vi "ntr.flow-panel.update.vi"(9 "log cluster":T5 {"clk" format="%#.3f"}, 11 "Controls[]":refnum<vi>[](array[refnum])) -> ()   [LabVIEW 2024]
uses:
  controls/typeEngineLogCluster.ctl
  controls/type.StepFunction.ctl
  controls/UiCompactReport.ctl
  controls/Ui.nrt.flow-panel.ctl
  controls/UiNutritionFlowElement.ctl
  controls/type.nrt.elment-state.ctl
  controls/enum-ntr-io-format.ctl
  controls/UiScheduleTimestamp.ctl
  controls/UiNutritionPanel.ctl
panel:
  out "Missing Element?":bool
  out "State(Element)":string
  out "Elements Names":string[](array[string])
  in  "Unit Settings":T1={"WASH_IN"={"boolean"=FALSE, "Message"="25/150"}, "EC"={"boolean"=TRUE, "Message"="L Alarm"}, "PH"={"boolean"=TRUE, "Message"="Low"}, "ORP"={"boolean"=TRUE, "Message"="Range"}, "W_TEMP"={"boolean"=TRUE, "Message"="25"}, "W_LEVEL"={"boolean"=TRUE, "Message"="FULL"}, "ALFA1"={"boolean"=TRUE, "Message"="60/60"}, "BETA1"={"boolean"=TRUE, "Message"="25/60"}, "ALFA2"={"boolean"=FALSE, "Message"="0/0"}, "BETA2"={"boolean"=FALSE, "Message"="0/0"}, "ACID"={"boolean"=FALSE, "Message"="0/60"}, "BASE"={"boolean"=FALSE, "Message"="0/50"}, "WATER"={"boolean"=FALSE, "Message"="0/150"}, "WASH_OUT"={"boolean"=FALSE, "Message"="ss"}, "UNIT"={"boolean"=FALSE, "Message"="25/150"}, "ORPMIX"={"boolean"=FALSE, "Message"="0/150"}}
  in  "TEST VECTOR":T3[](array[typedef])=[{"ErrorFlag"=FALSE, "idx"=0, "Step Name"="", "Step Function"=enum."UNIT_CHECK", "Report"="UNIT1:Prepare for Sampling", "clk"=808.9115753173828, "Proc"=""}, {"ErrorFlag"=FALSE, "idx"=1, "Step Name"="_START_UNIT", "Step Function"=enum."_IO_WRITE", "Report"="UNVLV_1;1:143,", "clk"=809.013774394989, "Proc"=""}, {"ErrorFlag"=FALSE, "idx"=2, "Step Name"="_AUX", "Step Function"=enum."_IO_WRITE", "Report"="UNPMP_1;1:143,", "clk"=809.1302719116211, "Proc"=""}, {"ErrorFlag"=FALSE, "idx"=3, "Step Name"="_WASH_IN", "Step Function"=enum."_DELAY_LOAD", "Report"="3807441809", "clk"=809.2404737472534, "Proc"=""}, {"ErrorFlag"=FALSE, "idx"=4, "Step Name"="", "Step Function"=enum."_DELAY_COMPARE", "Report"="2.0/2.0", "clk"=811.2761874198914, "Proc"=""}, {"ErrorFlag"=FALSE, "idx"=5, "Step Name"="", "Step Function"=enum."UNIT_SAMPLE", "Report"="UNIT=1;EC=2.7 LOW;PH=-38.0 ALARM;ORP=-38.0 ALARM;UNWL_1=0.0 LOW", "clk"=841.9652895927429, "Proc"=""}, {"ErrorFlag"=FALSE, "idx"=6, "Step Name"="", "Step Function"=enum."UNIT_DOSE", "Report"="pump=ALFA1;dose=2;counter=62;limit=200", "clk"=842.2391471862793, "Proc"=""}, {"ErrorFlag"=FALSE, "idx"=7, "Step Name"="_START_ALFA1", "Step Function"=enum."_IO_WRITE", "Report"="ALFA1;1:2,", "clk"=842.3526463508606, "Proc"=""}, {"ErrorFlag"=FALSE, "idx"=8, "Step Name"="_WAIT_ALFA1", "Step Function"=enum."_DELAY_LOAD", "Report"="3807441842", "clk"=842.4676065444946, "Proc"=""}, {"ErrorFlag"=FALSE, "idx"=9, "Step Name"="", "Step Function"=enum."_DELAY_COMPARE", "Report"="2.1/2.0", "clk"=844.5177793502808, "Proc"=""}, {"ErrorFlag"=FALSE, "idx"=10, "Step Name"="", "Step Function"=enum."UNIT_DOSE", "Report"="pump=BETA1;dose=2;counter=42;limit=100", "clk"=844.6215801239014, "Proc"=""}, {"ErrorFlag"=FALSE, "idx"=11, "Step Name"="_START_BETA1", "Step Function"=enum."_IO_WRITE", "Report"="BETA1;1:2,", "clk"=844.7354688644409, "Proc"=""}, {"ErrorFlag"=FALSE, "idx"=12, "Step Name"="_WAIT_BETA1", "Step Function"=enum."_DELAY_LOAD", "Report"="3807441845", "clk"=844.8503303527832, "Proc"=""}, {"ErrorFlag"=FALSE, "idx"=13, "Step Name"="", "Step Function"=enum."_DELAY_COMPARE", "Report"="2.1/2.0", "clk"=846.9136576652527, "Proc"=""}, {"ErrorFlag"=FALSE, "idx"=14, "Step Name"="", "Step Function"=enum."UNIT_DOSE", "Report"="pump=ALFA2;dose=3;counter=0;limit=20", "clk"=847.0166110992432, "Proc"=""}, {"ErrorFlag"=FALSE, "idx"=15, "Step Name"="_START_ALFA2", "Step Function"=enum."_IO_WRITE", "Report"="ALFA2;1:3,", "clk"=847.1284127235413, "Proc"=""}, {"ErrorFlag"=FALSE, "idx"=16, "Step Name"="_WAIT_ALFA2", "Step Function"=enum."_DELAY_LOAD", "Report"="3807441847", "clk"=847.2391495704651, "Proc"=""}, {"ErrorFlag"=FALSE, "idx"=17, "Step Name"="", "Step Function"=enum."_DELAY_COMPARE", "Report"="3.0/3.0", "clk"=850.2459425926208, "Proc"=""}, {"ErrorFlag"=FALSE, "idx"=18, "Step Name"="", "Step Function"=enum."UNIT_DOSE", "Report"="pump=BETA2;dose=3;counter=0;limit=20", "clk"=850.34832239151, "Proc"=""}, {"ErrorFlag"=FALSE, "idx"=19, "Step Name"="_START_BETA2", "Step Function"=enum."_IO_WRITE", "Report"="BETA2;1:3,", "clk"=850.4585151672363, "Proc"=""}, {"ErrorFlag"=FALSE, "idx"=20, "Step Name"="_WAIT_BETA2", "Step Function"=enum."_DELAY_LOAD", "Report"="3807441851", "clk"=850.5737953186035, "Proc"=""}, {"ErrorFlag"=FALSE, "idx"=21, "Step Name"="", "Step Function"=enum."_DELAY_COMPARE", "Report"="3.0/3.0", "clk"=853.5802583694458, "Proc"=""}, {"ErrorFlag"=FALSE, "idx"=22, "Step Name"="_WATER_AUX_OFF", "Step Function"=enum."_IO_WRITE", "Report"="UNPMP_1;0:0,", "clk"=853.6832575798035, "Proc"=""}, {"ErrorFlag"=FALSE, "idx"=23, "Step Name"="", "Step Function"=enum."UNIT_DOSE", "Report"="pump=WATER;dose=2;counter=20;limit=100", "clk"=853.7997298240662, "Proc"=""}, {"ErrorFlag"=FALSE, "idx"=24, "Step Name"="_START_WATER", "Step Function"=enum."_IO_WRITE", "Report"="WATER;1:2,", "clk"=853.9108262062073, "Proc"=""}, {"ErrorFlag"=FALSE, "idx"=25, "Step Name"="_WAIT_WATER", "Step Function"=enum."_DELAY_LOAD", "Report"="3807441854", "clk"=854.0239872932434, "Proc"=""}, {"ErrorFlag"=FALSE, "idx"=26, "Step Name"="", "Step Function"=enum."_DELAY_COMPARE", "Report"="2.1/2.0", "clk"=856.0921583175659, "Proc"=""}, {"ErrorFlag"=FALSE, "idx"=27, "Step Name"="_STOP_UNIT", "Step Function"=enum."_IO_WRITE", "Report"="UNVLV_1;0:0,", "clk"=856.1950078010559, "Proc"=""}, {"ErrorFlag"=FALSE, "idx"=28, "Step Name"="_AUX", "Step Function"=enum."_IO_WRITE", "Report"="UNPMP_1;0:0,", "clk"=856.3099999427795, "Proc"=""}, {"ErrorFlag"=FALSE, "idx"=29, "Step Name"="", "Step Function"=enum."UNIT_CHECK", "Report"="UNIT2:Unit Disabled", "clk"=856.4237542152405, "Proc"=""}, {"ErrorFlag"=FALSE, "idx"=30, "Step Name"="CYCLE_INTERVAL", "Step Function"=enum."_DELAY_LOAD", "Report"="3807441857", "clk"=856.5289416313171, "Proc"=""}, {"ErrorFlag"=FALSE, "idx"=31, "Step Name"="", "Step Function"=enum."_DELAY_COMPARE", "Report"="2.9/3.0", "clk"=859.4704394340515, "Proc"=""}] {"clk" format="%#.1f"}
  out "result string":string
  out "Step Name":string
  out "State":string
  in  "appended array":T5[](array[typedef])=[{"Proc Name"="NUTRITION", "ProcPath"="", "Step Name"="", "Step Function"=enum."_DELAY_COMPARE", "Step Index"=9, "Report"="1.5/3.0", "clk"=3806463695.106538, "error in"={"status"=FALSE, "code"=0, "source"=""}, "Log Message"="", "Proc Module"=""}, {"Proc Name"="NUTRITION", "ProcPath"="", "Step Name"="", "Step Function"=enum."_DELAY_COMPARE", "Step Index"=9, "Report"="0.8/3.0", "clk"=3806463694.341048, "error in"={"status"=FALSE, "code"=0, "source"=""}, "Log Message"="", "Proc Module"=""}, {"Proc Name"="NUTRITION", "ProcPath"="", "Step Name"="_WAIT_ALFA1", "Step Function"=enum."_DELAY_LOAD", "Step Index"=8, "Report"="", "clk"=3806463693.5845046, "error in"={"status"=FALSE, "code"=0, "source"=""}, "Log Message"="", "Proc Module"=""}, {"Proc Name"="NUTRITION", "ProcPath"="", "Step Name"="_AUX", "Step Function"=enum."_IO_WRITE", "Step Index"=7, "Report"="UNIT1,1:3,", "clk"=3806463692.8226175, "error in"={"status"=FALSE, "code"=0, "source"=""}, "Log Message"="", "Proc Module"=""}, {"Proc Name"="NUTRITION", "ProcPath"="", "Step Name"="_START_ALFA1", "Step Function"=enum."_IO_WRITE", "Step Index"=6, "Report"="ALFA1,1:3,", "clk"=3806463692.024861, "error in"={"status"=FALSE, "code"=0, "source"=""}, "Log Message"="", "Proc Module"=""}, {"Proc Name"="NUTRITION", "ProcPath"="", "Step Name"="", "Step Function"=enum."UNIT_DOSE", "Step Index"=5, "Report"="pump=ALFA1;dose=3;counter=3;limit=15", "clk"=3806463691.2188854, "error in"={"status"=FALSE, "code"=0, "source"=""}, "Log Message"="", "Proc Module"=""}, {"Proc Name"="NUTRITION", "ProcPath"="", "Step Name"="", "Step Function"=enum."UNIT_SAMPLE", "Step Index"=4, "Report"="UNIT=1;EC=5.0_LOW;PH=0.0_ALARM;ORP=-99;W_LEVEL=FULL;W_TEMP=25", "clk"=3806463690.4068866, "error in"={"status"=FALSE, "code"=0, "source"=""}, "Log Message"="", "Proc Module"=""}, {"Proc Name"="NUTRITION", "ProcPath"="", "Step Name"="", "Step Function"=enum."_DELAY_COMPARE", "Step Index"=3, "Report"="0.3/0.0", "clk"=3806463682.7784977, "error in"={"status"=FALSE, "code"=0, "source"=""}, "Log Message"="", "Proc Module"=""}, {"Proc Name"="NUTRITION", "ProcPath"="", "Step Name"="_WASH_IN", "Step Function"=enum."_DELAY_LOAD", "Step Index"=2, "Report"="", "clk"=3806463682.5215073, "error in"={"status"=FALSE, "code"=0, "source"=""}, "Log Message"="", "Proc Module"=""}, {"Proc Name"="NUTRITION", "ProcPath"="", "Step Name"="_START_FLOW", "Step Function"=enum."_IO_WRITE", "Step Index"=1, "Report"="UNIT1,1:5,", "clk"=3806463682.2498655, "error in"={"status"=FALSE, "code"=0, "source"=""}, "Log Message"="", "Proc Module"=""}, {"Proc Name"="NUTRITION", "ProcPath"="", "Step Name"="", "Step Function"=enum."UNIT_CHECK", "Step Index"=0, "Report"="UNIT1", "clk"=3806463681.9819593, "error in"={"status"=FALSE, "code"=0, "source"=""}, "Log Message"="", "Proc Module"=""}, {"Proc Name"="NUTRITION", "ProcPath"="", "Step Name"="", "Step Function"=enum."UNIT_CHECK", "Step Index"=0, "Report"="UNIT1", "clk"=3806457099.490219, "error in"={"status"=FALSE, "code"=0, "source"=""}, "Log Message"="", "Proc Module"=""}, {"Proc Name"="NUTRITION", "ProcPath"="", "Step Name"="_START_FLOW", "Step Function"=enum."_IO_WRITE", "Step Index"=1, "Report"="UNIT1,1:5,", "clk"=3806457099.753702, "error in"={"status"=FALSE, "code"=0, "source"=""}, "Log Message"="", "Proc Module"=""}, {"Proc Name"="NUTRITION", "ProcPath"="", "Step Name"="_WASH_IN", "Step Function"=enum."_DELAY_LOAD", "Step Index"=2, "Report"="", "clk"=3806457100.018482, "error in"={"status"=FALSE, "code"=0, "source"=""}, "Log Message"="", "Proc Module"=""}, {"Proc Name"="NUTRITION", "ProcPath"="", "Step Name"="", "Step Function"=enum."_DELAY_COMPARE", "Step Index"=3, "Report"="0.3/0.0", "clk"=3806457100.2720094, "error in"={"status"=FALSE, "code"=0, "source"=""}, "Log Message"="", "Proc Module"=""}, {"Proc Name"="NUTRITION", "ProcPath"="", "Step Name"="", "Step Function"=enum."UNIT_SAMPLE", "Step Index"=4, "Report"="UNIT=1;EC=5.0_LOW;PH=0.0_ALARM;ORP=-99;W_LEVEL=FULL;W_TEMP=25", "clk"=3806457100.531534, "error in"={"status"=FALSE, "code"=0, "source"=""}, "Log Message"="", "Proc Module"=""}, {"Proc Name"="NUTRITION", "ProcPath"="", "Step Name"="", "Step Function"=enum."UNIT_DOSE", "Step Index"=5, "Report"="ALFA1:3_0/15", "clk"=3806457100.830936, "error in"={"status"=FALSE, "code"=0, "source"=""}, "Log Message"="", "Proc Module"=""}, {"Proc Name"="NUTRITION", "ProcPath"="", "Step Name"="_START_ALFA1", "Step Function"=enum."_IO_WRITE", "Step Index"=6, "Report"="ALFA1,1:3,", "clk"=3806457101.096012, "error in"={"status"=FALSE, "code"=0, "source"=""}, "Log Message"="", "Proc Module"=""}, {"Proc Name"="NUTRITION", "ProcPath"="", "Step Name"="_AUX", "Step Function"=enum."_IO_WRITE", "Step Index"=7, "Report"="UNIT1,1:3,", "clk"=3806457101.359422, "error in"={"status"=FALSE, "code"=0, "source"=""}, "Log Message"="", "Proc Module"=""}, {"Proc Name"="NUTRITION", "ProcPath"="", "Step Name"="_WAIT_ALFA1", "Step Function"=enum."_DELAY_LOAD", "Step Index"=8, "Report"="", "clk"=3806457101.636155, "error in"={"status"=FALSE, "code"=0, "source"=""}, "Log Message"="", "Proc Module"=""}, {"Proc Name"="NUTRITION", "ProcPath"="", "Step Name"="", "Step Function"=enum."_DELAY_COMPARE", "Step Index"=9, "Report"="0.3/3.0", "clk"=3806457101.890099, "error in"={"status"=FALSE, "code"=0, "source"=""}, "Log Message"="", "Proc Module"=""}, {"Proc Name"="NUTRITION", "ProcPath"="", "Step Name"="", "Step Function"=enum."_DELAY_COMPARE", "Step Index"=9, "Report"="0.5/3.0", "clk"=3806457102.145725, "error in"={"status"=FALSE, "code"=0, "source"=""}, "Log Message"="", "Proc Module"=""}, {"Proc Name"="NUTRITION", "ProcPath"="", "Step Name"="", "Step Function"=enum."_DELAY_COMPARE", "Step Index"=9, "Report"="0.8/3.0", "clk"=3806457102.4017487, "error in"={"status"=FALSE, "code"=0, "source"=""}, "Log Message"="", "Proc Module"=""}, {"Proc Name"="NUTRITION", "ProcPath"="", "Step Name"="", "Step Function"=enum."_DELAY_COMPARE", "Step Index"=9, "Report"="1.0/3.0", "clk"=3806457102.662003, "error in"={"status"=FALSE, "code"=0, "source"=""}, "Log Message"="", "Proc Module"=""}, {"Proc Name"="NUTRITION", "ProcPath"="", "Step Name"="", "Step Function"=enum."_DELAY_COMPARE", "Step Index"=9, "Report"="1.3/3.0", "clk"=3806457102.9161887, "error in"={"status"=FALSE, "code"=0, "source"=""}, "Log Message"="", "Proc Module"=""}, {"Proc Name"="NUTRITION", "ProcPath"="", "Step Name"="", "Step Function"=enum."_DELAY_COMPARE", "Step Index"=9, "Report"="1.5/3.0", "clk"=3806457103.1737394, "error in"={"status"=FALSE, "code"=0, "source"=""}, "Log Message"="", "Proc Module"=""}, {"Proc Name"="NUTRITION", "ProcPath"="", "Step Name"="", "Step Function"=enum."_DELAY_COMPARE", "Step Index"=9, "Report"="1.8/3.0", "clk"=3806457103.4284744, "error in"={"status"=FALSE, "code"=0, "source"=""}, "Log Message"="", "Proc Module"=""}, {"Proc Name"="NUTRITION", "ProcPath"="", "Step Name"="", "Step Function"=enum."_DELAY_COMPARE", "Step Index"=9, "Report"="2.0/3.0", "clk"=3806457103.683892, "error in"={"status"=FALSE, "code"=0, "source"=""}, "Log Message"="", "Proc Module"=""}, {"Proc Name"="NUTRITION", "ProcPath"="", "Step Name"="", "Step Function"=enum."_DELAY_COMPARE", "Step Index"=9, "Report"="2.3/3.0", "clk"=3806457103.9400506, "error in"={"status"=FALSE, "code"=0, "source"=""}, "Log Message"="", "Proc Module"=""}, {"Proc Name"="NUTRITION", "ProcPath"="", "Step Name"="", "Step Function"=enum."_DELAY_COMPARE", "Step Index"=9, "Report"="2.6/3.0", "clk"=3806457104.203483, "error in"={"status"=FALSE, "code"=0, "source"=""}, "Log Message"="", "Proc Module"=""}, {"Proc Name"="NUTRITION", "ProcPath"="", "Step Name"="", "Step Function"=enum."_DELAY_COMPARE", "Step Index"=9, "Report"="2.8/3.0", "clk"=3806457104.4665594, "error in"={"status"=FALSE, "code"=0, "source"=""}, "Log Message"="", "Proc Module"=""}, {"Proc Name"="NUTRITION", "ProcPath"="", "Step Name"="", "Step Function"=enum."_DELAY_COMPARE", "Step Index"=9, "Report"="3.1/3.0", "clk"=3806457104.722045, "error in"={"status"=FALSE, "code"=0, "source"=""}, "Log Message"="", "Proc Module"=""}, {"Proc Name"="NUTRITION", "ProcPath"="", "Step Name"="", "Step Function"=enum."UNIT_DOSE", "Step Index"=10, "Report"="BETA1:3_0/15", "clk"=3806457104.9829454, "error in"={"status"=FALSE, "code"=0, "source"=""}, "Log Message"="", "Proc Module"=""}, {"Proc Name"="NUTRITION", "ProcPath"="", "Step Name"="_START_BETA1", "Step Function"=enum."_IO_WRITE", "Step Index"=11, "Report"="BETA1,1:3,", "clk"=3806457105.259259, "error in"={"status"=FALSE, "code"=0, "source"=""}, "Log Message"="", "Proc Module"=""}, {"Proc Name"="NUTRITION", "ProcPath"="", "Step Name"="_AUX", "Step Function"=enum."_IO_WRITE", "Step Index"=12, "Report"="UNIT1,1:3,", "clk"=3806457105.5364633, "error in"={"status"=FALSE, "code"=0, "source"=""}, "Log Message"="", "Proc Module"=""}, {"Proc Name"="NUTRITION", "ProcPath"="", "Step Name"="_WAIT_BETA1", "Step Function"=enum."_DELAY_LOAD", "Step Index"=13, "Report"="", "clk"=3806457105.8045793, "error in"={"status"=FALSE, "code"=0, "source"=""}, "Log Message"="", "Proc Module"=""}, {"Proc Name"="NUTRITION", "ProcPath"="", "Step Name"="", "Step Function"=enum."_DELAY_COMPARE", "Step Index"=14, "Report"="0.3/3.0", "clk"=3806457106.0651937, "error in"={"status"=FALSE, "code"=0, "source"=""}, "Log Message"="", "Proc Module"=""}, {"Proc Name"="NUTRITION", "ProcPath"="", "Step Name"="", "Step Function"=enum."_DELAY_COMPARE", "Step Index"=14, "Report"="0.5/3.0", "clk"=3806457106.321509, "error in"={"status"=FALSE, "code"=0, "source"=""}, "Log Message"="", "Proc Module"=""}] {"clk" format="%#.3f"}
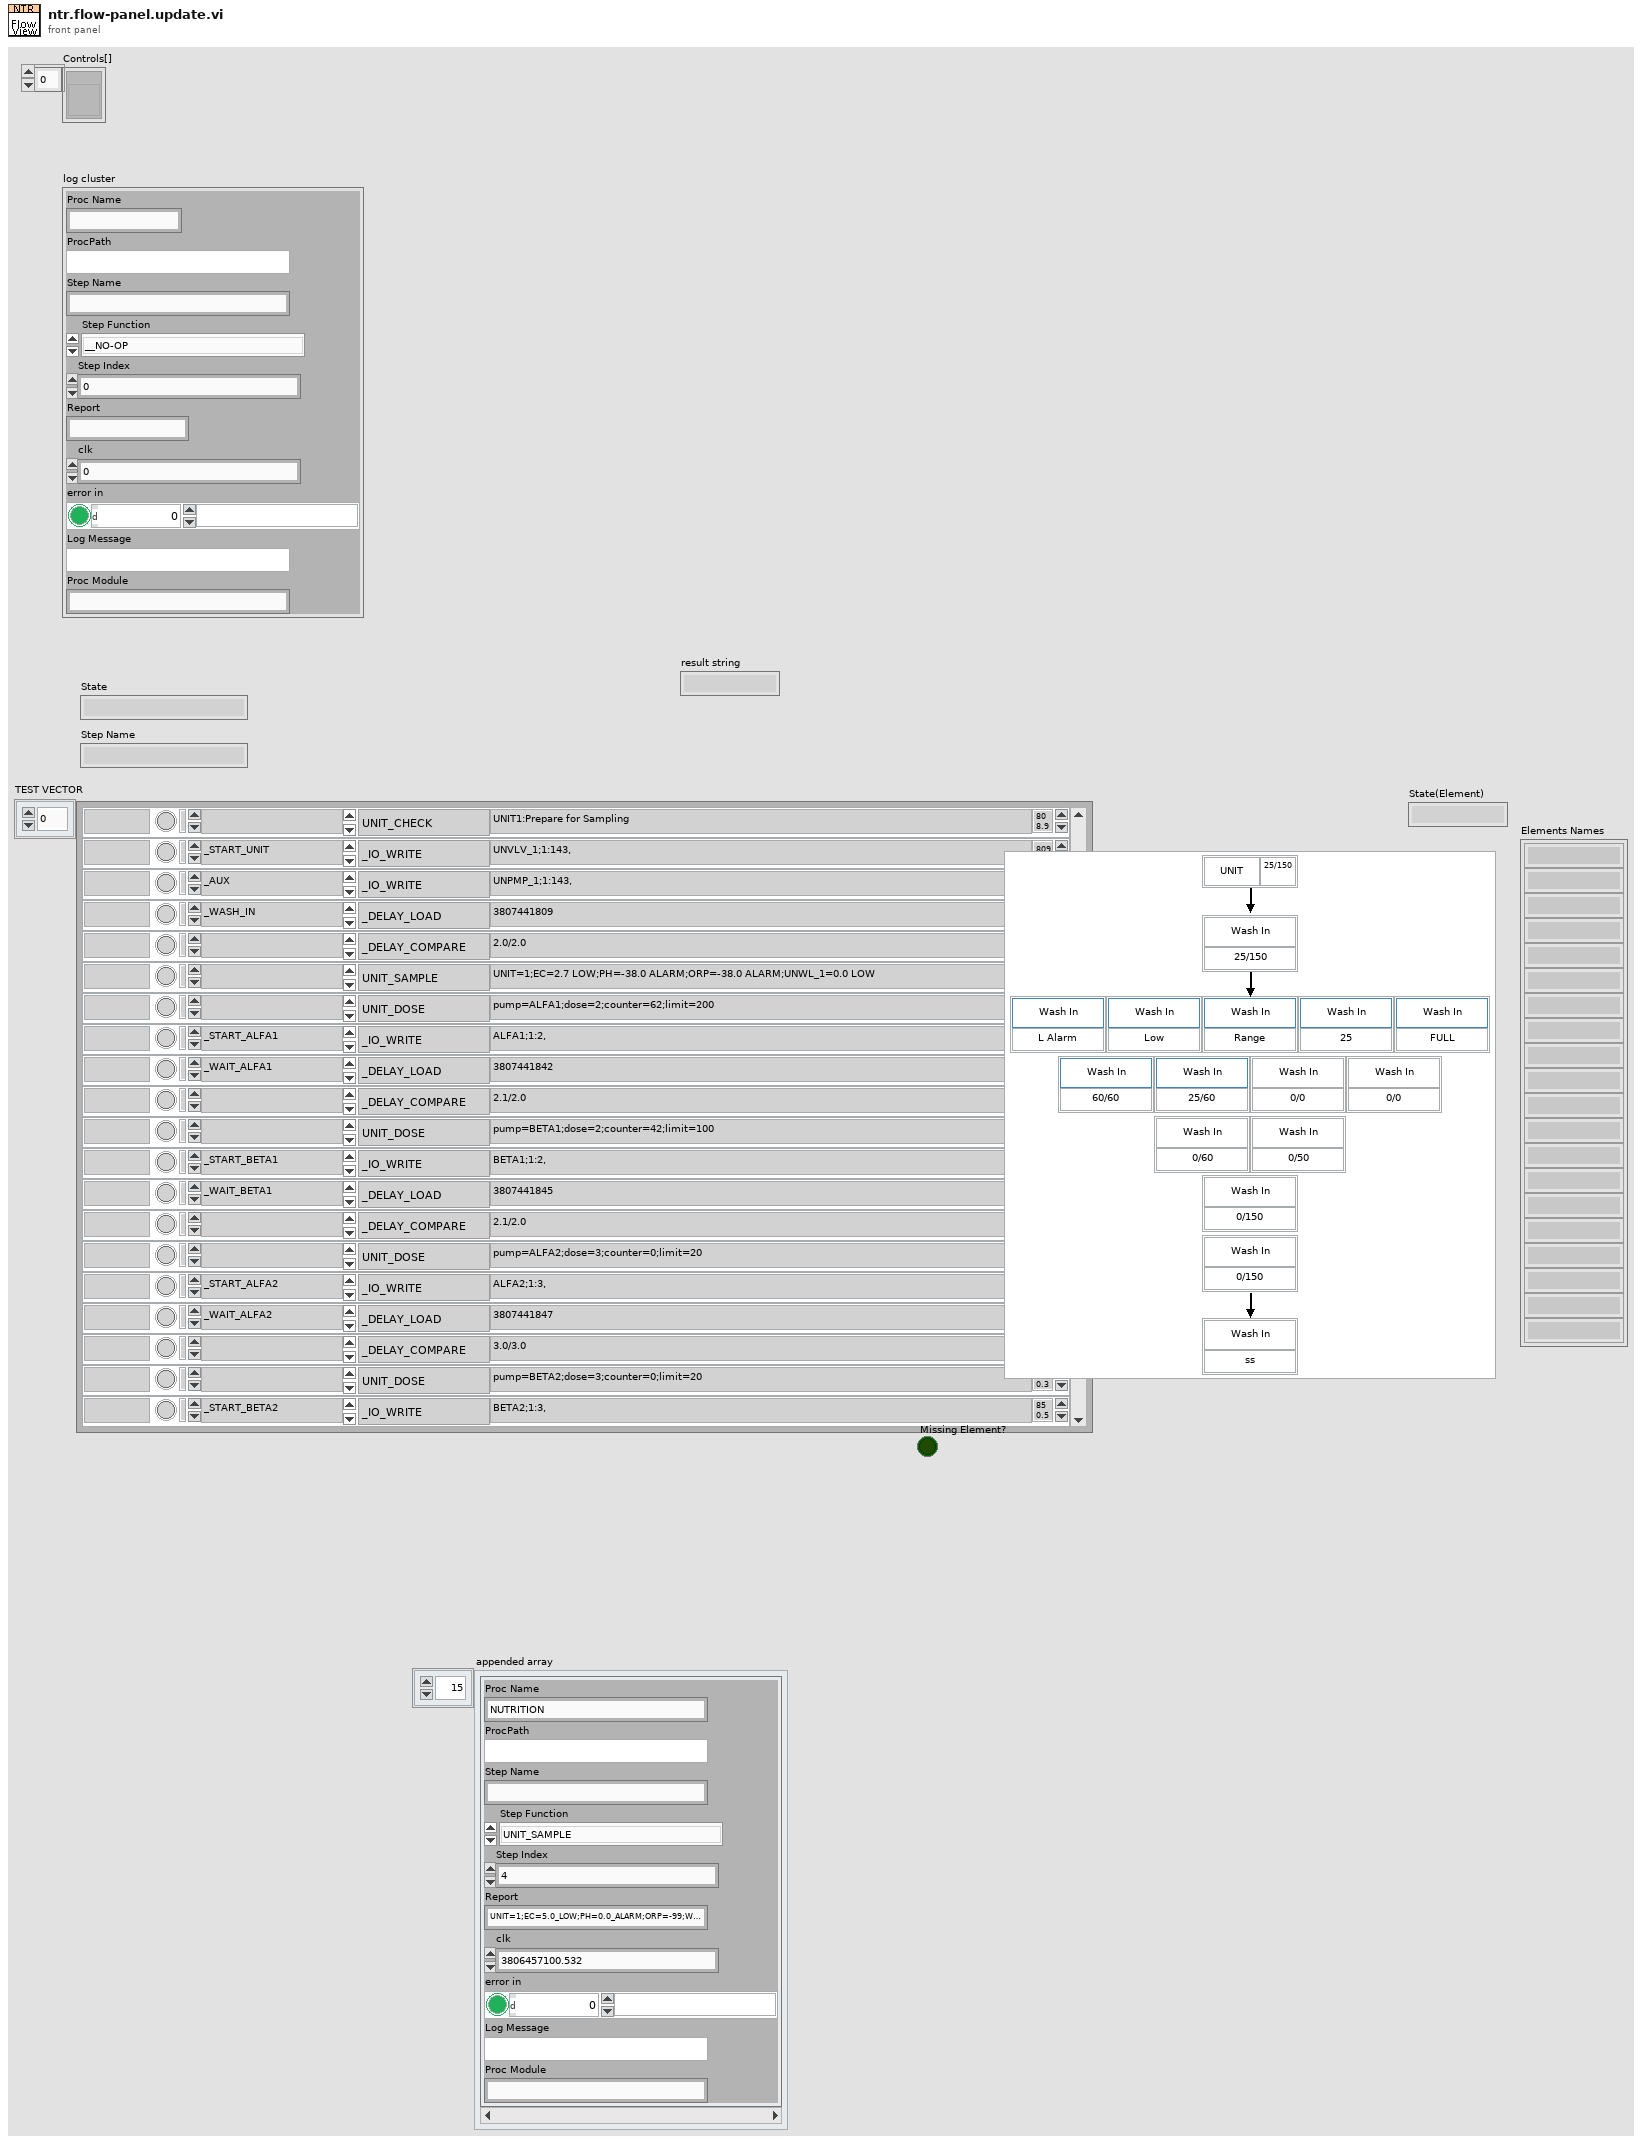
[diagram p1: front panel]
types:
  T1 = typedef "Ui.nrt.flow-panel.ctl" = cluster{"WASH_IN":T2, "EC":T2, "PH":T2, "ORP":T2, "W_TEMP":T2, "W_LEVEL":T2, "ALFA1":T2, "BETA1":T2, "ALFA2":T2, "BETA2":T2, "ACID":T2, "BASE":T2, "WATER":T2, "WASH_OUT":T2, "UNIT":cluster{"boolean":bool, "Message":string}, "ORPMIX":T2}
  T2 = typedef "UiNutritionFlowElement.ctl" = cluster{"boolean":bool, "Message":string}
  T3 = typedef "UiCompactReport.ctl" = cluster{"ErrorFlag":bool, "idx":i32, "Step Name":string, "Step Function":T4, "Report":string, "clk":dbl, "Proc":string}
  T4 = typedef "type.StepFunction.ctl" = enum16{"__NO-OP", "_DELAY_LOAD", "_DELAY_COMPARE", "_JUMP", "_COMPLETE", "_COMPARE", "_LOG_MESSAGE", "_LOG_LAST_REPORT", "_SCHEDULE", "_SCHED_DAILY", "CLK_COMPARE", "PROC_START", "PROC_STOP", "PROC_LOAD", "PROC_COMPLETION_CHECK", "PROC_COMPLETION_LOAD", "_IO_READ", "_IO_READ_MANY", "_IO_WRITE", "_IO_WRITE_BY_REG", "_IO_GET_OUTPUT", "_OCS_CHECK", "_OCS_RECORD", "_GET_RH", "_GET_ACC_UV", "_GET_WD", "_GET_WS", "_REC_DELETE", "_REC_MOVE", "_REC_COPY", "_IRR_CHECK", "UNIT_CHECK", "UNIT_SAMPLE", "UNIT_DOSE"}
  T5 = typedef "typeEngineLogCluster.ctl" = cluster{"Proc Name":string, "ProcPath":string, "Step Name":string, "Step Function":T4, "Step Index":i32, "Report":string, "clk":dbl, "error in":errorcluster, "Log Message":string, "Proc Module":string}
  T6 = typedef "type.nrt.elment-state.ctl" = enum16{"No Change", "OFF", "In Range", "Out of Range", "Alarm"}
  T7 = typedef "UiNutritionPanel.ctl" = cluster{"Main":cluster{"Enable":bool, "WashTimes":cluster{"In":dbl, "Out":dbl}, "DailyActivityHours":cluster{"Begin Time":T8, "End Time":T8}[]}, "Water Dosing":cluster{"Water Dose":dbl, "Water Limit":dbl}, "EC Ranges":cluster{"H Alarm":dbl, "L Alarm":dbl, "Low":dbl}, "EC Dosing":cluster{"ALFA1 Dose":dbl, "ALFA1 Limit":dbl, "BETA1 Dose":dbl, "BETA1 Limit":dbl, "ALFA2 Dose":dbl, "ALFA2 Limit":dbl, "BETA2 Dose":dbl, "BETA2 Limit":dbl}, "PH Ranges":cluster{"H Alarm":dbl, "L Alarm":dbl, "High":dbl, "Low":dbl}, "PH Dosing":cluster{"ACID Dose":dbl, "ACID Limit":dbl, "BASE Dose":dbl, "BASE Limit":dbl}, "ORP Ranges":cluster{"H Alarm":dbl, "L Alarm":dbl, "Low":dbl}, "ORP Dosing":cluster{"MIX Dose":dbl, "MIX Limit":dbl}}
  T8 = typedef "UiScheduleTimestamp.ctl" = timestamp
  T9 = typedef "enum-ntr-io-format.ctl" = enum16{"UN_VLV%d", "UN_PMP%d", "UN_WL%d", "UN_PH", "UN_EC", "UN_ORP", "UN_WT", "UN_PH2", "UN_ALFA1", "UN_BETA1", "UN_ALFA2", "UN_BETA2", "UN_ACID", "UN_BASE", "UN_WATER", "UN_ORPMIX"}
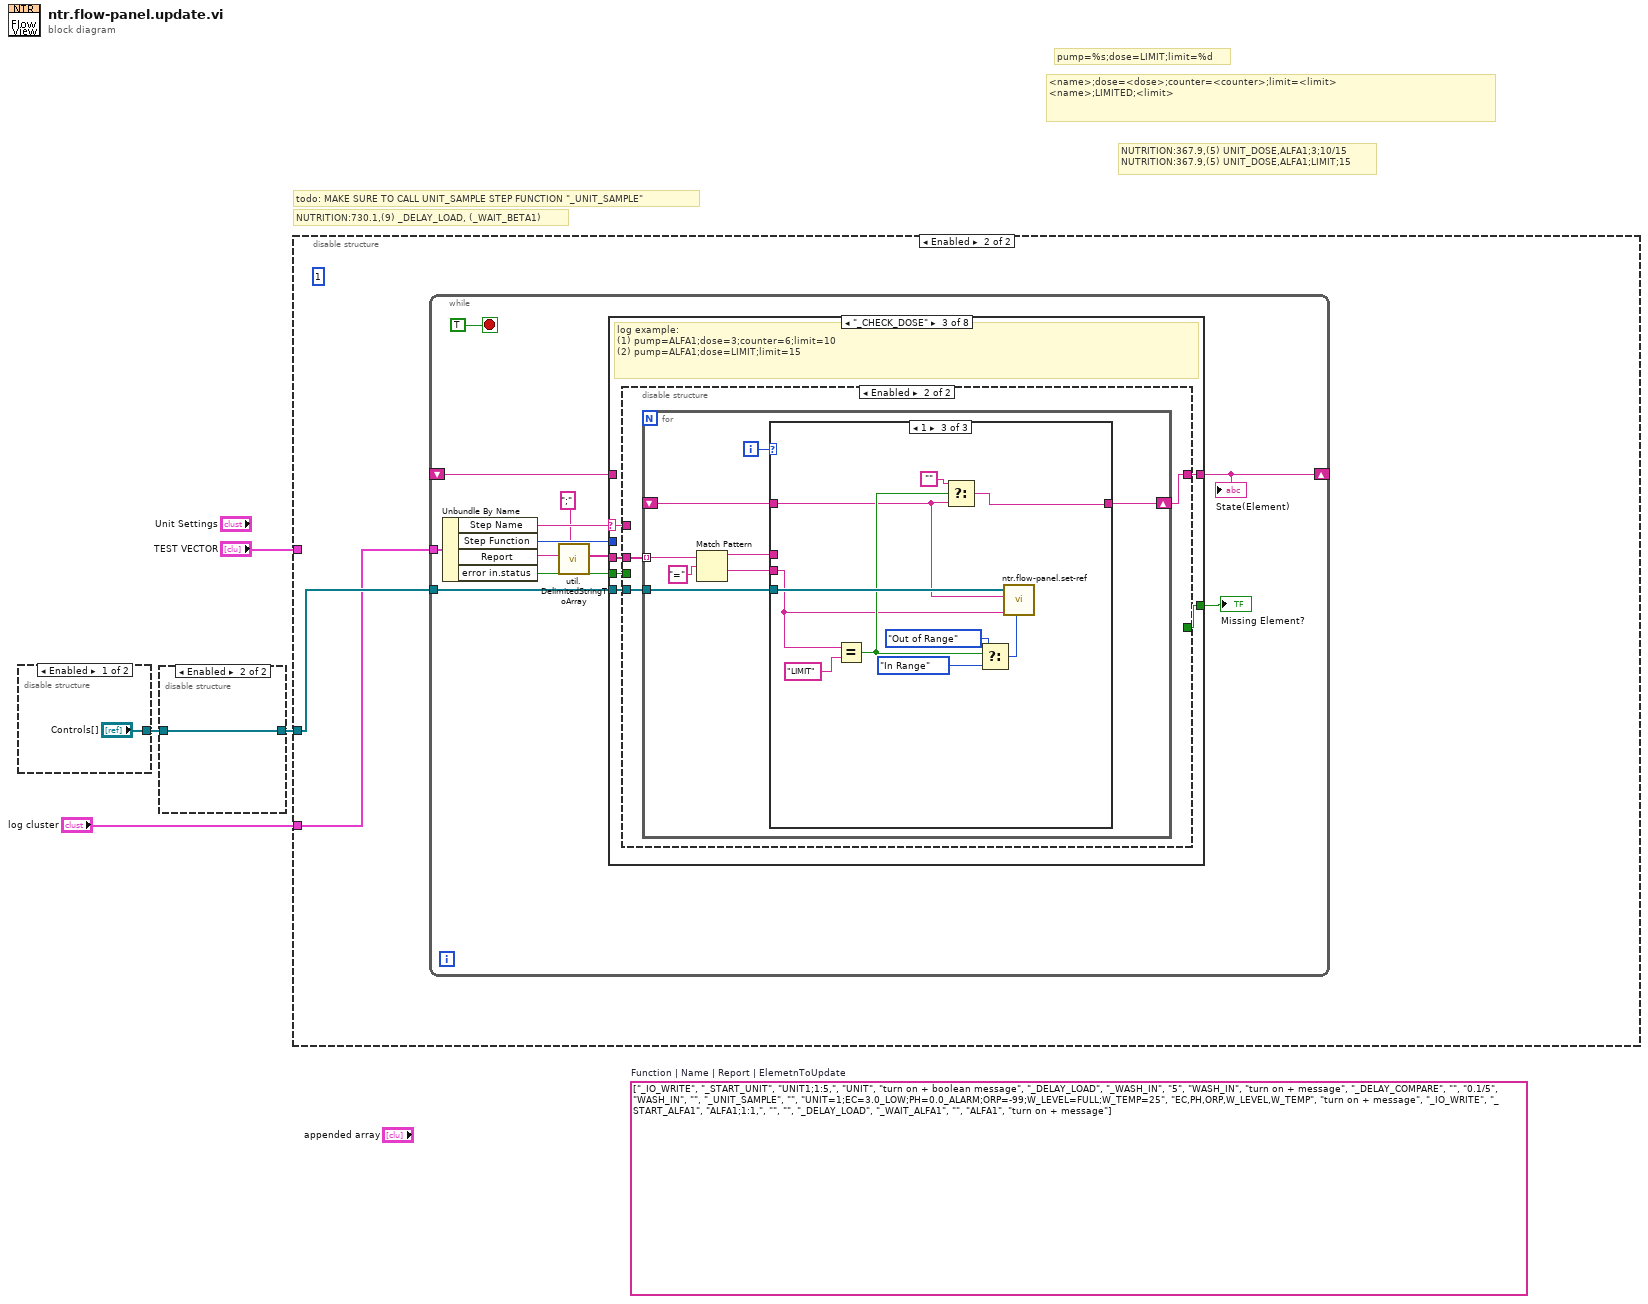
[diagram p0: block diagram]
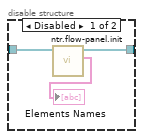
[diagram p2: hidden frame]
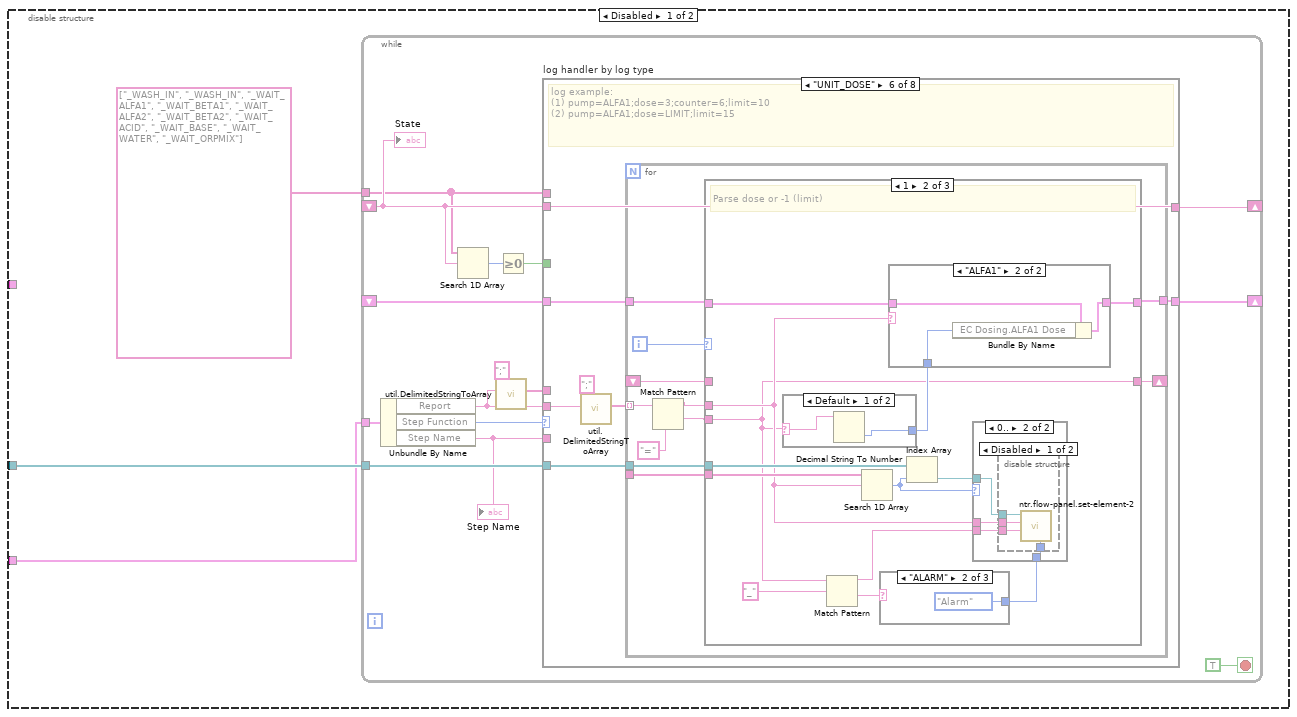
[diagram p3: hidden frame]
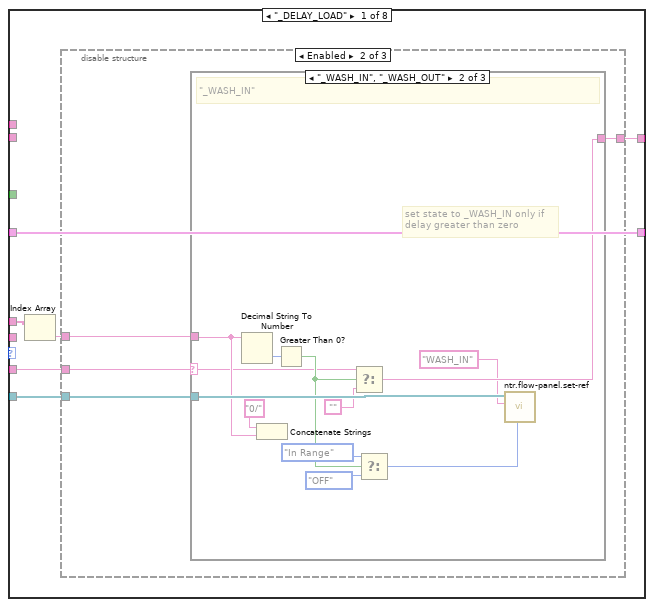
[diagram p4: hidden frame]
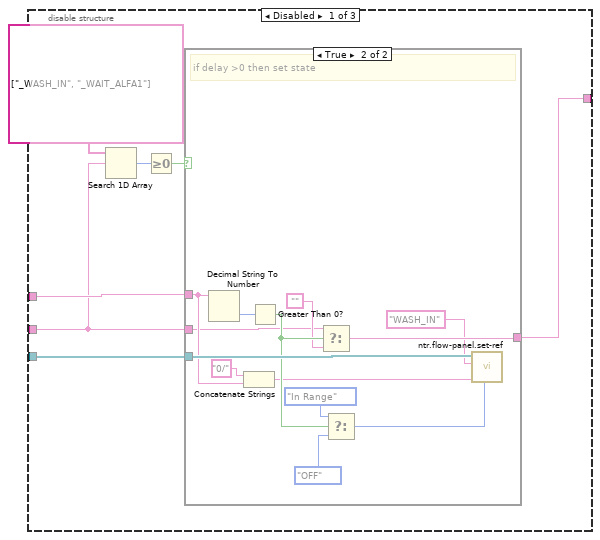
[diagram p5: hidden frame]
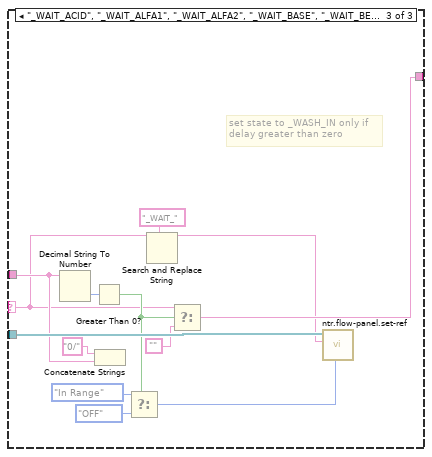
[diagram p8: hidden frame]
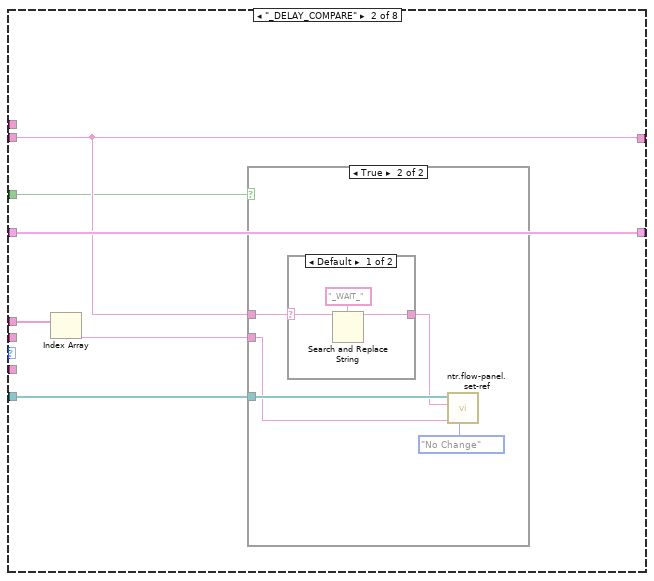
[diagram p10: hidden frame]
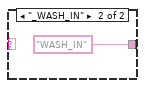
[diagram p12: hidden frame]
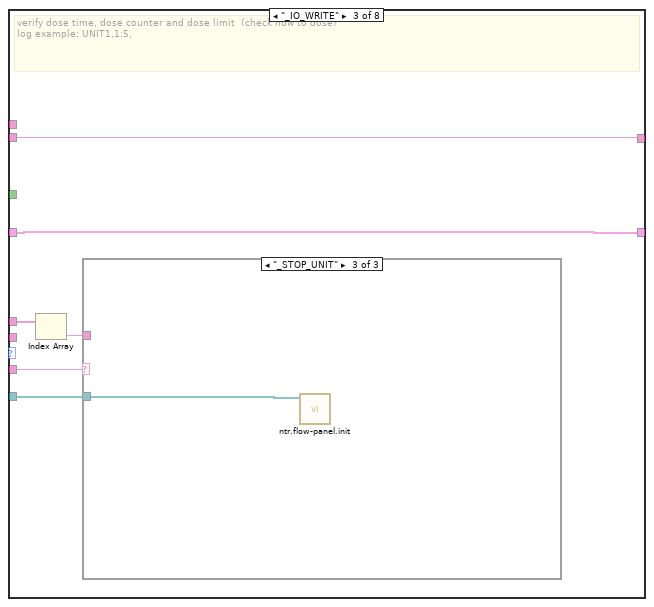
[diagram p13: hidden frame]
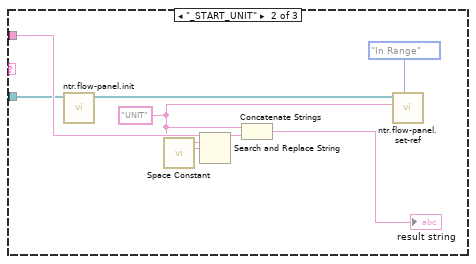
[diagram p15: hidden frame]
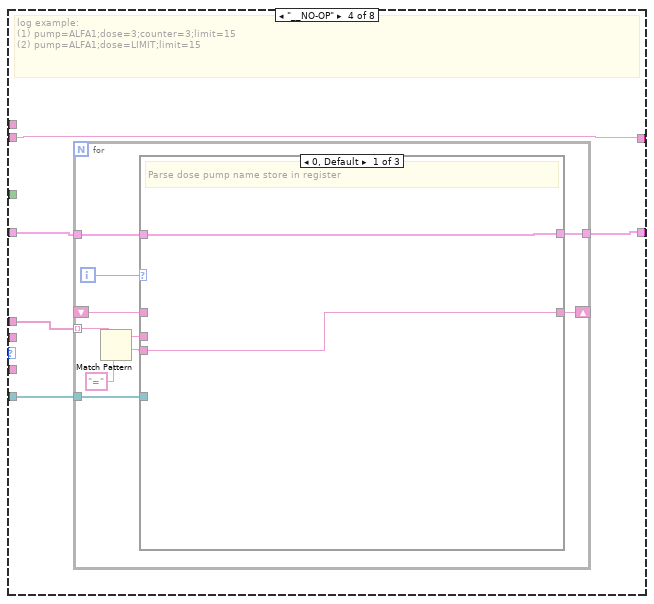
[diagram p16: hidden frame]
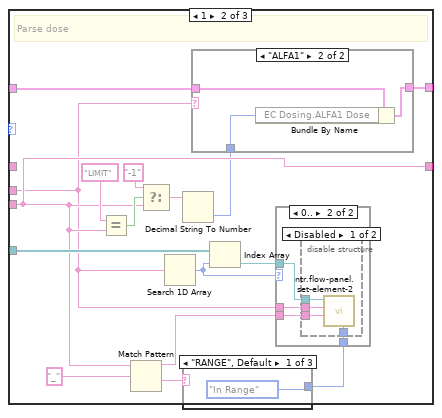
[diagram p17: hidden frame]
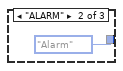
[diagram p19: hidden frame]
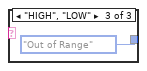
[diagram p20: hidden frame]
diagram:
  (unwired) string[][] [["_IO_WRITE", "_START_UNIT", "UNIT1;1:5,", "UNIT", "turn on + boolean message"], ["_DELAY_LOAD", "_WASH_IN", "5", "WASH_IN", "turn on + message"], ["_DELAY_COMPARE", "", "0.1/5", "WASH_IN", ""], ["_UNIT_SAMPLE", "", "UNIT=1;EC=3.0_LOW;PH=0.0_ALARM;ORP=-99;W_LEVEL=FULL;W_TEMP=25", "EC,PH,ORP,W_LEVEL,W_TEMP", "turn on + message"], ["_IO_WRITE", "_START_ALFA1", "ALFA1;1:1,", "", ""], ["_DELAY_LOAD", "_WAIT_ALFA1", "", "ALFA1", "turn on + message"]]  # Function | Name | Report | ElemetnToUpdate
  # "todo: MAKE SURE TO CALL UNIT_SAMPLE STEP FUNCTION \"_UNIT_SAMPLE\""
  # "pump=%s;dose=LIMIT;limit=%d"
  # "NUTRITION:367.9,(5) UNIT_DOSE,ALFA1;3;10/15\nNUTRITION:367.9,(5) UNIT_DOSE,ALFA1;LIMIT;15"
  # "<name>;dose=<dose>;counter=<counter>;limit=<limit>\n<name>;LIMITED;<limit>"
  # "NUTRITION:730.1,(9) _DELAY_LOAD, (_WAIT_BETA1)"
  n1 = disable-structure shown="Enabled" {
    disable-tunnel: ["Controls[]" w6] -> w4
    frame Enabled {
    }
    frame Disabled {
      n2 = property on="Unit Settings" class="Clust (strict)"() -> ("Controls[]"=w6:refnum<vi>[])  [unwired: 2 in, 2 out]
    }
  }
  n3 = disable-structure shown="Enabled" {
    disable-tunnel: w4 -> [w9 w10]
    disable-tunnel: [w8 w10] -> w3
    frame Disabled {
      n4 = call "ntr.flow-panel.init.vi"("Controls in"=w9) -> ("Elements Names"=→"Elements Names":string[], "Controls out"=w8:refnum<vi>[])  [unwired: 8 in, 1 out]
    }
    frame Enabled {
    }
  }
  n5 = disable-structure shown="Enabled" {
    disable-tunnel: w3 -> [w13 w281]
    disable-tunnel: "TEST VECTOR" -> [_ _]
    disable-tunnel: "log cluster" -> [w11 w280]
    frame Disabled {
      n6 = while {
        tunnel: w13 -> [w28]
        tunnel: w11 -> [w27]
        shift-right: [w23] -> _
        shift-left: _ -> [w22]
        shift-right: [w18] -> _
        shift-left: _ -> [w17]
        tunnel: string[] ["_WASH_IN", "_WASH_IN", "_WAIT_ALFA1", "_WAIT_BETA1", "_WAIT_ALFA2", "_WAIT_BETA2", "_WAIT_ACID", "_WAIT_BASE", "_WAIT_WATER", "_WAIT_ORPMIX"] ("Element Name") -> [w14]
        stop <- TRUE stop-if-true
        n7 = Unbundle By Name(w27) -> ("Report"=w20:string, "Step Function"=w26:T4, "Step Name"=w25:string)
        "Step Name" <- w25
        n8 = Search 1D Array(1D array=w14, element=w17) -> (index of element=w16:i32)  [unwired: 1 in]
        n9 = call "util.DelimitedStringToArray.vi"("delimiter (,)"=";", "delimitaed string"=w20) -> ("array out"=w19:string[])  [unwired: 9 in]
        n10 = Greater Or Equal To 0?(x=w16) -> (x >= 0?=w15:bool)
        n11 = case "log handler by log type" shown="\"UNIT_DOSE\"" w26 {
          tunnel: w20 -> [_ _ _ _ _ w199 _ _]
          tunnel: w28 -> [w33 w88 w104 w118 _ w201 w264 _]
          tunnel: w25 -> [w29 _ w103 _ _ _ _ _]
          tunnel: [w34 w89 w102 w116 T7 {"Main"={"Enable"=FALSE, "WashTimes"={"In"=0.0, "Out"=0.0}, "DailyActivityHours"=[]}, "Water Dosing"={"Water Dose"=0.0, "Water Limit"=0.0}, "EC Ranges"={"H Alarm"=0.0, "L Alarm"=0.0, "Low"=0.0}, "EC Dosing"={"ALFA1 Dose"=0.0, "ALFA1 Limit"=0.0, "BETA1 Dose"=0.0, "BETA1 Limit"=0.0, "ALFA2 Dose"=0.0, "ALFA2 Limit"=0.0, "BETA2 Dose"=0.0, "BETA2 Limit"=0.0}, "PH Ranges"={"H Alarm"=10.0, "L Alarm"=3.0, "High"=0.0, "Low"=6.0}, "PH Dosing"={"ACID Dose"=3.0, "ACID Limit"=15.0, "BASE Dose"=3.0, "BASE Limit"=15.0}, "ORP Ranges"={"H Alarm"=0.0, "L Alarm"=0.0, "Low"=0.0}, "ORP Dosing"={"MIX Dose"=0.0, "MIX Limit"=0.0}} ("Cluster") w197 w263 w279] -> w23
          tunnel: w22 -> [w34 w89 w102 w117 _ w198 w263 w279]
          tunnel: w19 -> [w32 w87 w101 w115 _ _ w261 _]
          tunnel: [w30 w85 w100 w114 "" w196 w262 w278] -> w18
          tunnel: w17 -> [_ w85 w100 w114 _ w196 w262 w278]
          tunnel: w15 -> [_ w84 _ _ _ _ _ _]
          tunnel: w14 -> [_ _ _ _ _ _ _ _]
          frame "_DELAY_LOAD" {
            n12 = Index Array(array=w32) -> (element=w31:string)  [unwired: 1 in]
            n13 = disable-structure shown="Enabled" {
              disable-tunnel: w33 -> [w41 w58 _]
              disable-tunnel: w31 -> [w40 w57 _]
              disable-tunnel: [w39 w56 _] -> w30
              disable-tunnel: w29 -> [w35 w55 _]
              frame Disabled {
                n14 = Search 1D Array(1D array=string[] ["_WASH_IN", "_WAIT_ALFA1"] ("Element Name"), element=w35) -> (index of element=w37:i32)  [unwired: 1 in]
                n15 = Greater Or Equal To 0?(x=w37) -> (x >= 0?=w36:bool)
                n16 = case shown="True" w36 {
                  tunnel: w41 -> [_ w54]
                  tunnel: w40 -> [_ w43]
                  tunnel: [_ w51] -> w39
                  tunnel: w35 -> [_ w42]
                  frame False {
                  }
                  frame True {
                    # "if delay >0 then set state"
                    n17 = Decimal String To Number(string=w43) -> (number=w53:i32)  [unwired: 2 in, 1 out]
                    n18 = Concatenate Strings("0/" ("string"), w43) -> (w44:string)
                    n19 = Greater Than 0?(x=w53) -> (x > 0?=w52:bool)
                    n20 = Select(t=w42, s=w52, f="") -> (s? t:f=w51:string)
                    n21 = Select(t=type.nrt.elment-state."In Range" ("Enum 2"), s=w52, f=type.nrt.elment-state."OFF" ("Enum 2")) -> (s? t:f=w46:T6)
                    n22 = call "ntr.flow-panel.set-ref.vi"("Enum"=w46, "String Message"=w44, "Element Name"="WASH_IN", "refs"=w54) -> ()  [unwired: 7 in, 1 out]
                  }
                }
              }
              frame Enabled {
                n23 = case shown="\"_WASH_IN\", \"_WASH_OUT\"" w55 {
                  selector: w55 -> [_ w59 w73]
                  tunnel: w58 -> [_ w70 w83]
                  tunnel: w57 -> [_ w69 w82]
                  tunnel: [_ w68 w81] -> w56
                  frame Default {
                    # "reset state when _DELAY is ignored (Default case)"
                  }
                  frame "_WASH_IN", "_WASH_OUT" {
                    # "set state to _WASH_IN only if\ndelay greater than zero"
                    # "\"_WASH_IN\""
                    n24 = Decimal String To Number(string=w69) -> (number=w67:i32)  [unwired: 2 in, 1 out]
                    n25 = Concatenate Strings("0/" ("string"), w69) -> ()  [unwired: 1 out]
                    n26 = Greater Than 0?(x=w67) -> (x > 0?=w66:bool)
                    n27 = Select(t=w59, s=w66, f="") -> (s? t:f=w68:string)
                    n28 = Select(t=type.nrt.elment-state."In Range" ("Enum 2"), s=w66, f=type.nrt.elment-state."OFF" ("Enum 2")) -> (s? t:f=w61:T6)
                    n29 = call "ntr.flow-panel.set-ref.vi"("Enum"=w61, "Element Name"="WASH_IN", "refs"=w70) -> ()  [unwired: 8 in, 1 out]
                  }
                  frame "_WAIT_ACID", "_WAIT_ALFA1", "_WAIT_ALFA2", "_WAIT_BASE", "_WAIT_BETA1", "_WAIT_BETA2", "_WAIT_WATER" {
                    # "set state to _WASH_IN only if\ndelay greater than zero"
                    n30 = Decimal String To Number(string=w82) -> (number=w80:i32)  [unwired: 2 in, 1 out]
                    n31 = Greater Than 0?(x=w80) -> (x > 0?=w79:bool)
                    n32 = Concatenate Strings("0/" ("string"), w82) -> ()  [unwired: 1 out]
                    n33 = Select(t=type.nrt.elment-state."In Range" ("Enum 2"), s=w79, f=type.nrt.elment-state."OFF" ("Enum 2")) -> (s? t:f=w75:T6)
                    n34 = Search and Replace String(input string=w73, search string="_WAIT_") -> (result string=w71:string)  [unwired: 6 in, 3 out]
                    n35 = Select(t=w73, s=w79, f="") -> (s? t:f=w81:string)
                    n36 = call "ntr.flow-panel.set-ref.vi"("Enum"=w75, "Element Name"=w71, "refs"=w83) -> ()  [unwired: 8 in, 1 out]
                  }
                }
              }
              frame Disabled {
              }
            }
          }
          frame "_DELAY_COMPARE" {
            n37 = Index Array(array=w87) -> (element=w86:string)  [unwired: 1 in]
            n38 = case shown="True" w84 {
              tunnel: w88 -> [_ w94]
              tunnel: w86 -> [_ w92]
              tunnel: w85 -> [_ w90]
              frame False {
              }
              frame True {
                n39 = case shown="Default" w90 {
                  selector: w90 -> [w96 _]
                  tunnel: [w95 "WASH_IN" ("Element Name")] -> w91
                  frame Default {
                    n40 = Search and Replace String(input string=w96, search string="_WAIT_") -> (result string=w95:string)  [unwired: 6 in, 3 out]
                  }
                  frame "_WASH_IN" {
                  }
                }
                n41 = call "ntr.flow-panel.set-ref.vi"("Enum"=type.nrt.elment-state."No Change", "String Message"=w92, "Element Name"=w91, "refs"=w94) -> ()  [unwired: 7 in, 1 out]
              }
            }
          }
          frame "_IO_WRITE" {
            # "verify dose time, dose counter and dose limit  (check how to dose)\nlog example: UNIT1,1:5,"
            n42 = Index Array(array=w101) -> (element=w99:string)  [unwired: 1 in]
            n43 = case shown="\"_STOP_UNIT\"" w103 {
              tunnel: w104 -> [_ w105 w113]
              tunnel: w99 -> [_ w109 _]
              frame Default {
              }
              frame "_START_UNIT" {
                w107 = "UNIT" ("search string/char (-)")
                n44 = call "ntr.flow-panel.init.vi"("Controls in"=w105) -> ("Controls out"=w106:refnum<vi>[])  [unwired: 8 in, 2 out]
                n45 = call <vilib>:"Space Constant.vi"() -> ("String"=w111:string)
                n46 = Search and Replace String(input string=w109, search string=w107, replace string=w111) -> (result string=w110:string)  [unwired: 5 in, 3 out]
                n47 = Concatenate Strings(w107, w110) -> (→"result string":string)
                n48 = call "ntr.flow-panel.set-ref.vi"("Enum"=type.nrt.elment-state."In Range" ("Enum 2"), "Element Name"=w107, "refs"=w106) -> ()  [unwired: 8 in, 1 out]
              }
              frame "_STOP_UNIT" {
                n49 = call "ntr.flow-panel.init.vi"("Controls in"=w113) -> ()  [unwired: 8 in, 3 out]
              }
            }
          }
          frame "__NO-OP" {
            # "log example: \n(1) pump=ALFA1;dose=3;counter=3;limit=15\n(2) pump=ALFA1;dose=LIMIT;limit=15"
            n50 = for {
              tunnel: w115 -> [w127] mode=indexing
              tunnel: w118 -> [w126]
              tunnel: w117 -> [w125]
              tunnel: [w124] -> w116
              shift-right: [w119] -> _
              shift-left: _ -> [w121]
              i -> [w123]
              n51 = Match Pattern(string=w127, regular expression="=") -> (after substring=w120:string)  [unwired: 1 in, 3 out]
              n52 = case shown="0, Default" w123 {
                tunnel: w127 -> [_ w130 w162]
                tunnel: w126 -> [_ w145 w177]
                tunnel: w125 -> [w129 w138 w170]
                tunnel: [w129 w137 w169] -> w124
                tunnel: w120 -> [w128 w133 w165]
                tunnel: w121 -> [_ _ _]
                tunnel: [w128 w133 w165] -> w119
                frame 0, Default {
                  # "Parse dose pump name store in register"
                }
                frame 1 {
                  # "Parse dose"
                  n53 = Equal?(x="LIMIT" ("y"), y=w133) -> (x = y?=w136:bool)
                  n54 = Match Pattern(string=w133, regular expression="_") -> (before substring=w139:string, after substring=w140:string)  [unwired: 1 in, 2 out]
                  n55 = Select(t="-1" ("y"), s=w136, f=w133) -> (s? t:f=w132:string)
                  n56 = Search 1D Array(element=w130) -> (1D array=w146:string[], index of element=w143:i32)  [unwired: 1 in]
                  n57 = Decimal String To Number(string=w132) -> (number=w131:i32)  [unwired: 2 in, 1 out]
                  n58 = case shown="\"RANGE\", Default" w140 {
                    tunnel: [enum16{"In Range", "Out of Range", "Alarm"}."In Range" ("Enum") enum16{"In Range", "Out of Range", "Alarm"}."Alarm" ("Enum") enum16{"In Range", "Out of Range", "Alarm"}."Out of Range" ("Enum")] -> w142
                    frame "RANGE", Default {
                    }
                    frame "ALARM" {
                    }
                    frame "HIGH", "LOW" {
                    }
                  }
                  n59 = case shown="\"ALFA1\"" w130 {
                    tunnel: w138 -> [w147 w150]
                    tunnel: [w147 w149] -> w137
                    tunnel: w131 -> [_ w148]
                    frame "False", Default {
                    }
                    frame "ALFA1" {
                      n60 = Bundle By Name(cluster=w150, "EC Dosing.ALFA1 Dose"=w148) -> (w149:T7)
                    }
                  }
                  n61 = Index Array(array=w145, index=w143) -> (element=w144:refnum<vi>)
                  n62 = case shown="0.." w143 {
                    tunnel: w144 -> [_ w157]
                    tunnel: w130 -> [_ w156]
                    tunnel: w139 -> [_ w155]
                    tunnel: w142 -> [_ w154]
                    frame ..-1, Default {
                    }
                    frame 0.. {
                      n63 = disable-structure shown="Disabled" {
                        disable-tunnel: w157 -> [w161 _]
                        disable-tunnel: w156 -> [w160 _]
                        disable-tunnel: w155 -> [w159 _]
                        disable-tunnel: w154 -> [w158 _]
                        frame Disabled {
                          n64 = call "ntr.flow-panel.set-element-2.vi"("Enum 2"=w158, "Message Text"=w159, "Boolean Text (empty: no change)"=w160, "Ctl Refnum"=w161) -> ()  [unwired: 7 in, 1 out]
                        }
                        frame Enabled {
                        }
                      }
                    }
                  }
                }
                frame 2 {
                  # "Parse limit"
                  n65 = Equal?(x="LIMIT" ("y"), y=w165) -> (x = y?=w168:bool)
                  n66 = Match Pattern(string=w165, regular expression="_") -> (before substring=w171:string, after substring=w172:string)  [unwired: 1 in, 2 out]
                  n67 = Select(t="-1" ("y"), s=w168, f=w165) -> (s? t:f=w164:string)
                  n68 = Search 1D Array(element=w162) -> (1D array=w178:string[], index of element=w175:i32)  [unwired: 1 in]
                  n69 = Decimal String To Number(string=w164) -> (number=w163:i32)  [unwired: 2 in, 1 out]
                  n70 = case shown="\"RANGE\", Default" w172 {
                    tunnel: [enum16{"In Range", "Out of Range", "Alarm"}."In Range" ("Enum") enum16{"In Range", "Out of Range", "Alarm"}."Alarm" ("Enum") enum16{"In Range", "Out of Range", "Alarm"}."Out of Range" ("Enum")] -> w174
                    frame "RANGE", Default {
                    }
                    frame "ALARM" {
                    }
                    frame "HIGH", "LOW" {
                    }
                  }
                  n71 = case shown="\"False\", Default" w162 {
                    tunnel: w170 -> [w179 w182]
                    tunnel: [w179 w181] -> w169
                    tunnel: w163 -> [_ w180]
                    frame "False", Default {
                    }
                    frame "ALFA1" {
                      n72 = Bundle By Name(cluster=w182, "EC Dosing.ALFA1 Dose"=w180) -> (w181:T7)
                    }
                  }
                  n73 = Index Array(array=w177, index=w175) -> (element=w176:refnum<vi>)
                  n74 = case shown="0.." w175 {
                    tunnel: w176 -> [_ w189]
                    tunnel: w162 -> [_ w188]
                    tunnel: w171 -> [_ w187]
                    tunnel: w174 -> [_ w186]
                    frame ..-1, Default {
                    }
                    frame 0.. {
                      n75 = disable-structure shown="Disabled" {
                        disable-tunnel: w189 -> [w193 _]
                        disable-tunnel: w188 -> [w192 _]
                        disable-tunnel: w187 -> [w191 _]
                        disable-tunnel: w186 -> [w190 _]
                        frame Disabled {
                          n76 = call "ntr.flow-panel.set-element-2.vi"("Enum 2"=w190, "Message Text"=w191, "Boolean Text (empty: no change)"=w192, "Ctl Refnum"=w193) -> ()  [unwired: 7 in, 1 out]
                        }
                        frame Enabled {
                        }
                      }
                    }
                  }
                }
              }
            }
          }
          frame "UNIT_CHECK" {
            # "initialize"
          }
          frame "UNIT_DOSE" {
            # "log example: \n(1) pump=ALFA1;dose=3;counter=6;limit=10\n(2) pump=ALFA1;dose=LIMIT;limit=15"
            n77 = call "util.DelimitedStringToArray.vi"("delimiter (,)"=";", "delimitaed string"=w199) -> ("array out"=w202:string[])  [unwired: 9 in]
            n78 = for {
              tunnel: w202 -> [w214] mode=indexing
              tunnel: w201 -> [w212]
              tunnel: [w213] -> w200
              tunnel: w198 -> [w211]
              tunnel: [w210] -> w197
              shift-right: [w205] -> _
              shift-left: _ -> [w207]
              i -> [w209]
              n79 = Match Pattern(string=w214, regular expression="=") -> (before substring=w204:string, after substring=w206:string)  [unwired: 1 in, 2 out]
              n80 = case shown="1" w209 {
                tunnel: w204 -> [_ w219 w249]
                tunnel: w213 -> [_ w229 _]
                tunnel: w212 -> [_ w228 w248]
                tunnel: w211 -> [w216 w222 w253]
                tunnel: [w216 w221 w252] -> w210
                tunnel: w206 -> [w215 w217 w251]
                tunnel: w207 -> [_ _ w250]
                tunnel: [w215 w217 w250] -> w205
                frame 0, Default {
                  # "Parse dosepump name"
                }
                frame 1 {
                  # "Parse dose or -1 (limit)"
                  n81 = case shown="Default" w217 {
                    selector: w217 -> [w231 _]
                    tunnel: [w230 -1] -> w220
                    frame Default {
                      n82 = Decimal String To Number(string=w231) -> (number=w230:i32)  [unwired: 2 in, 1 out]
                    }
                    frame "LIMIT" {
                    }
                  }
                  n83 = Match Pattern(string=w217, regular expression="_") -> (before substring=w223:string, after substring=w224:string)  [unwired: 1 in, 2 out]
                  n84 = Search 1D Array(1D array=w229, element=w219) -> (index of element=w226:i32)  [unwired: 1 in]
                  n85 = case shown="\"ALARM\"" w224 {
                    tunnel: [type.nrt.elment-state."In Range" ("Enum 2") type.nrt.elment-state."Alarm" ("Enum 2") type.nrt.elment-state."Out of Range" ("Enum 2")] -> w218
                    frame "RANGE", Default {
                    }
                    frame "ALARM" {
                    }
                    frame "HIGH", "LOW" {
                    }
                  }
                  n86 = case shown="\"ALFA1\"" w219 {
                    tunnel: w222 -> [w233 w236]
                    tunnel: [w233 w235] -> w221
                    tunnel: w220 -> [_ w234]
                    frame "False", Default {
                    }
                    frame "ALFA1" {
                      n87 = Bundle By Name(cluster=w236, "EC Dosing.ALFA1 Dose"=w234) -> (w235:T7)
                    }
                  }
                  n88 = Index Array(array=w228, index=w226) -> (element=w227:refnum<vi>)
                  n89 = case shown="0.." w226 {
                    tunnel: w227 -> [_ w243]
                    tunnel: w219 -> [_ w242]
                    tunnel: w223 -> [_ w241]
                    tunnel: w218 -> [_ w240]
                    frame ..-1, Default {
                    }
                    frame 0.. {
                      n90 = disable-structure shown="Disabled" {
                        disable-tunnel: w243 -> [w247 _]
                        disable-tunnel: w242 -> [w246 _]
                        disable-tunnel: w241 -> [w245 _]
                        disable-tunnel: w240 -> [w244 _]
                        frame Disabled {
                          n91 = call "ntr.flow-panel.set-element-2.vi"("Enum 2"=w244, "Message Text"=w245, "Boolean Text (empty: no change)"=w246, "Ctl Refnum"=w247) -> ()  [unwired: 7 in, 1 out]
                        }
                        frame Enabled {
                        }
                      }
                    }
                  }
                }
                frame 2 {
                  # "Parse limit"
                  n92 = case shown="\"limit\"" w249 {
                    tunnel: w253 -> [w254 w260]
                    tunnel: [w254 w260] -> w252
                    tunnel: w251 -> [_ w255]
                    tunnel: w250 -> [_ w259]
                    tunnel: w248 -> [_ w258]
                    frame "False", Default {
                    }
                    frame "limit" {
                      # "if limit"
                      n93 = Format Into String(format string="LIMIT(%s)" ("String Message"), w255) -> (resulting string=w256:string)  [unwired: 2 in, 1 out]
                      n94 = call "ntr.flow-panel.set-ref.vi"(9:w256, "Element Name"=w259, "refs"=w258) -> ()  [unwired: 8 in, 1 out]
                    }
                  }
                }
              }
            }
          }
          frame "UNIT_SAMPLE" {
            # "\"UNIT_SAMPLE\" \nparse report\nlog example:\nUNIT=1;EC=5.0_RANGE;PH=0.0_ALARM;ORP=-99;W_LEVEL=FULL;W_TEMP=25"
            n95 = for {
              tunnel: w261 -> [w274] mode=indexing
              tunnel: w264 -> [w272]
              n96 = Match Pattern(string=w274, regular expression="=") -> (before substring=w269:string, after substring=w273:string)  [unwired: 1 in, 2 out]
              n97 = Match Pattern(string=w273, regular expression="_") -> (before substring=w267:string, after substring=w266:string)  [unwired: 1 in, 2 out]
              n98 = case shown="\"HIGH\", \"LOW\"" w266 {
                tunnel: [type.nrt.elment-state."In Range" ("Enum") type.nrt.elment-state."Alarm" ("Enum 2") type.nrt.elment-state."Out of Range" ("Enum")] -> w265
                frame "RANGE", Default {
                }
                frame "ALARM" {
                }
                frame "HIGH", "LOW" {
                }
              }
              n99 = call <vilib>:"Space Constant.vi"() -> ("String"=w268:string)
              n100 = Concatenate Strings(w269, w268, w267) -> ()  [unwired: 1 out]
              n101 = call "ntr.flow-panel.set-ref.vi"("Enum"=w265, "String Message"=w266, "Element Name"=w269, "refs"=w272) -> ()  [unwired: 7 in, 1 out]
            }
          }
          frame Default {
          }
        }
        "State" <- w17
      }
    }
    frame Enabled {
      (unwired) 1
      n102 = while {
        tunnel: w280 -> [w292]
        tunnel: w281 -> [w290]
        shift-right: [w289] -> _
        shift-left: _ -> [w288]
        stop <- TRUE stop-if-true
        n103 = Unbundle By Name(w292) -> ("Step Name"=w291:string, "Step Function"=w287:T4, "Report"=w284:string, "error in.status"=w286:bool)
        n104 = call "util.DelimitedStringToArray.vi"("delimiter (,)"=";", "delimitaed string"=w284) -> ("array out"=w283:string[])  [unwired: 9 in]
        n105 = case shown="\"_CHECK_DOSE\"" w291 {
          selector: w291 -> [_ _ w329 w428 w435 _ w508 _]
          tunnel: w290 -> [w298 w315 w334 w417 w430 w451 w517 _]
          tunnel: [w294 w312 w331 w428 w435 "WASH_IN" w506 w518] -> w289
          tunnel: w288 -> [w294 w312 _ _ _ _ _ w518]
          tunnel: w287 -> [w295 _ _ _ _ _ _ _]
          tunnel: w283 -> [w296 w313 w332 w423 w433 w449 w512 _]
          tunnel: w286 -> [w297 w314 w333 w427 w434 w450 w516 _]
          tunnel: [_ _ w330 w419 w432 w447 _ _] -> w282
          frame "" {
            # "nameless step (check step function)"
            n106 = case shown="\"_DELAY_COMPARE\"" w295 {
              tunnel: w298 -> [_ w306 w311]
              tunnel: w297 -> [_ w300 _]
              tunnel: w296 -> [_ w302 _]
              tunnel: w294 -> [_ w299 _]
              frame Default {
              }
              frame "_DELAY_COMPARE" {
                n107 = Index Array(array=w302) -> (element=w301:string)  [unwired: 1 in]
                n108 = Select(t=type.nrt.elment-state."Alarm" ("Enum"), s=w300, f=type.nrt.elment-state."In Range" ("Enum")) -> (s? t:f=w303:T6)
                n109 = case shown="Default" w299 {
                  tunnel: w306 -> [_ w310]
                  tunnel: w303 -> [_ w309]
                  tunnel: w299 -> [_ w308]
                  tunnel: w301 -> [_ w307]
                  frame "" {
                    # "empty state - bypass element update"
                  }
                  frame Default {
                    n110 = call "ntr.flow-panel.set-ref.vi"("Enum"=w309, "String Message"=w307, "Element Name"=w308, "refs"=w310) -> ()  [unwired: 7 in, 1 out]
                  }
                }
              }
              frame "UNIT_CHECK" {
                n111 = call "ntr.flow-panel.init.vi"("Controls in"=w311) -> ()  [unwired: 8 in, 3 out]
              }
            }
          }
          frame "_AUX" {
            n112 = case shown="\"_START_UNIT\"" w312 {
              tunnel: w315 -> [_ w318]
              tunnel: w314 -> [_ w317]
              tunnel: w313 -> [_ w316]
              frame "False", Default {
              }
              frame "_START_UNIT" {
                n113 = disable-structure shown="Enabled" {
                  disable-tunnel: w318 -> [w327 _]
                  disable-tunnel: w317 -> [w326 _]
                  disable-tunnel: w316 -> [w322 _]
                  frame Disabled {
                    n114 = Index Array(array=w322) -> (element=w321:string)  [unwired: 1 in]
                    n115 = Match Pattern(string=w321, regular expression="_") -> (after substring=w319:string)  [unwired: 1 in, 3 out]
                    n116 = Select(t=type.nrt.elment-state."Alarm" ("Enum"), s=w326, f=type.nrt.elment-state."In Range" ("Enum")) -> (s? t:f=w323:T6)
                    n117 = call "ntr.flow-panel.set-ref.vi"("Enum"=w323, "String Message"=w319, "Element Name"="UNIT", "refs"=w327) -> ()  [unwired: 7 in, 1 out]
                  }
                  frame Enabled {
                  }
                }
              }
            }
          }
          frame "_CHECK_DOSE" {
            # "log example: \n(1) pump=ALFA1;dose=3;counter=6;limit=10\n(2) pump=ALFA1;dose=LIMIT;limit=15"
            n118 = disable-structure shown="Enabled" {
              disable-tunnel: w334 -> [w339 w395]
              disable-tunnel: w333 -> [w338 _]
              disable-tunnel: w332 -> [w337 w396]
              disable-tunnel: ["WASH_IN" w394] -> w331
              disable-tunnel: [w335 _] -> w330
              disable-tunnel: w329 -> [_ _]
              frame Disabled {
                n119 = for {
                  tunnel: w339 -> [w347]
                  tunnel: w338 -> [w346]
                  tunnel: w337 -> [w345] mode=indexing
                  tunnel: [w344] -> w335
                  n120 = Match Pattern(string=w345, regular expression="=") -> (before substring=w341:string, after substring=w342:string)  [unwired: 1 in, 2 out]
                  n121 = case shown="Default" w341 {
                    selector: w341 -> [w348 w362]
                    tunnel: w347 -> [w357 w371]
                    tunnel: w346 -> [w356 w370]
                    tunnel: [w355 w369] -> w344
                    tunnel: w342 -> [w349 w363]
                    tunnel: string[] ["UNWL", "UNWT"] ("regular expression") -> [_ w361]
                    frame "EC", "ORP", "PH" {
                      n122 = call <vilib>:"Space Constant.vi"() -> ("String"=w351:string)
                      n123 = Match Pattern(string=w349, regular expression=w351) -> (after substring=w352:string)  [unwired: 1 in, 3 out]
                      n124 = case shown="\"ALARM\"" w352 {
                        tunnel: [type.nrt.elment-state."In Range" ("Enum 2") type.nrt.elment-state."Alarm" ("Enum 2") type.nrt.elment-state."Out of Range" ("Enum 2")] -> w350
                        frame "RANGE", Default {
                        }
                        frame "ALARM" {
                        }
                        frame "HIGH", "LOW" {
                        }
                      }
                      n125 = Select(t=type.nrt.elment-state."Alarm" ("Enum"), s=w356, f=w350) -> (s? t:f=w353:T6)
                      n126 = call "ntr.flow-panel.set-ref.vi"("Enum"=w353, "String Message"=w349, "Element Name"=w348, "refs"=w357) -> ("Missing Element? (error)"=w355:bool)  [unwired: 7 in]
                    }
                    frame Default {
                      n127 = call <vilib>:"Space Constant.vi"() -> ("String"=w365:string)
                      n128 = Match Pattern(string=w363, regular expression=w365) -> (after substring=w366:string)  [unwired: 1 in, 3 out]
                      n129 = case shown="\"HIGH\", \"LOW\"" w366 {
                        tunnel: [type.nrt.elment-state."In Range" ("Enum 2") type.nrt.elment-state."Alarm" ("Enum 2") type.nrt.elment-state."Out of Range" ("Enum 2")] -> w364
                        frame "RANGE", Default {
                        }
                        frame "ALARM" {
                        }
                        frame "HIGH", "LOW" {
                        }
                      }
                      n130 = Select(t=type.nrt.elment-state."Alarm" ("Enum"), s=w370, f=w364) -> (s? t:f=w367:T6)
                      n131 = for {
                        tunnel: w371 -> [w380]
                        tunnel: [w379] -> w369
                        tunnel: w367 -> [w378]
                        tunnel: w363 -> [w374]
                        tunnel: w362 -> [w377]
                        tunnel: w361 -> [w376] mode=indexing
                        n132 = call <vilib>:"Space Constant.vi"() -> ("String"=w373:string)
                        n133 = Match Pattern(string=w374, regular expression=w373) -> (after substring=w372:string)  [unwired: 1 in, 3 out]
                        n134 = Match Pattern(string=w377, regular expression=w376) -> (match substring=w375:string)  [unwired: 1 in, 3 out]
                        n135 = case shown="\"UNWL\"" w375 {
                          tunnel: w380 -> [_ w385 w390]
                          tunnel: [_ w384 w389] -> w379
                          tunnel: w378 -> [_ w383 w388]
                          tunnel: w374 -> [_ _ w387]
                          tunnel: w372 -> [_ w381 _]
                          frame "0", Default {
                          }
                          frame "UNWL" {
                            n136 = call "ntr.flow-panel.set-ref.vi"("Enum"=w383, "String Message"=w381, "Element Name"="W_LEVEL", "refs"=w385) -> ("Missing Element? (error)"=w384:bool)  [unwired: 7 in]
                          }
                          frame "UNWT" {
                            n137 = call "ntr.flow-panel.set-ref.vi"("Enum"=w388, "String Message"=w387, "Element Name"="W_TEMP", "refs"=w390) -> ("Missing Element? (error)"=w389:bool)  [unwired: 7 in]
                          }
                        }
                      }
                    }
                  }
                }
              }
              frame Enabled {
                n138 = for {
                  tunnel: w396 -> [w402] mode=indexing
                  tunnel: w395 -> [w404]
                  shift-right: [w398] -> w394
                  shift-left: _ -> [w397]
                  i -> [w403]
                  n139 = Match Pattern(string=w402, regular expression="=") -> (before substring=w400:string, after substring=w399:string)  [unwired: 1 in, 2 out]
                  n140 = case shown="1" w403 {
                    tunnel: w404 -> [_ _ w416]
                    tunnel: w400 -> [_ _ _]
                    tunnel: w399 -> [_ w406 w409]
                    tunnel: [w405 w406 w408] -> w398
                    tunnel: w397 -> [w405 _ w407]
                    frame -1, Default {
                    }
                    frame 0 {
                      # "get 1st param (Dose pump name)"
                    }
                    frame 1 {
                      n141 = Equal?(x=w409, y="LIMIT") -> (x = y?=w411:bool)
                      n142 = Select(t="", s=w411, f=w407) -> (s? t:f=w408:string)
                      n143 = Select(t=type.nrt.elment-state."Out of Range" ("Enum"), s=w411, f=type.nrt.elment-state."In Range" ("Enum")) -> (s? t:f=w412:T6)
                      n144 = call "ntr.flow-panel.set-ref.vi"("Enum"=w412, "String Message"=w409, "Element Name"=w407, "refs"=w416) -> ()  [unwired: 7 in, 1 out]
                    }
                  }
                }
              }
            }
          }
          frame "_START_UNIT" {
            (unwired) enum-ntr-io-format."UN_VLV%d"
            # "UN_VLV5;1:128,"
            n145 = Index Array(array=w423) -> (element=w422:string)  [unwired: 1 in]
            n146 = call "ntr.flow-panel.init.vi"("Controls in"=w417) -> ("Controls out"=w418:refnum<vi>[])  [unwired: 8 in, 2 out]
            n147 = Match Pattern(string=w422, regular expression="UN_VLV") -> (after substring=w420:string)  [unwired: 1 in, 3 out]
            n148 = Select(t=type.nrt.elment-state."Alarm" ("Enum"), s=w427, f=type.nrt.elment-state."In Range" ("Enum")) -> (s? t:f=w424:T6)
            n149 = call "ntr.flow-panel.set-ref.vi"("Enum"=w424, "String Message"=w420, "Element Name"="UNIT", "refs"=w418) -> ("Missing Element? (error)"=w419:bool)  [unwired: 7 in]
          }
          frame "_STOP_UNIT" {
            n150 = call "ntr.flow-panel.init.vi"("Controls in"=w430) -> ("Controls out"=w431:refnum<vi>[])  [unwired: 8 in, 2 out]
            n151 = disable-structure shown="Enabled" {
              disable-tunnel: w434 -> [w445 _]
              disable-tunnel: w433 -> [w441 _]
              disable-tunnel: [w437 _] -> w432
              disable-tunnel: w431 -> [w436 _]
              frame Disabled {
                n152 = Index Array(array=w441) -> (element=w440:string)  [unwired: 1 in]
                n153 = Match Pattern(string=w440, regular expression="_") -> (after substring=w438:string)  [unwired: 1 in, 3 out]
                n154 = Select(t=type.nrt.elment-state."Alarm" ("Enum"), s=w445, f=type.nrt.elment-state."In Range" ("Enum")) -> (s? t:f=w442:T6)
                n155 = call "ntr.flow-panel.set-ref.vi"("Enum"=w442, "String Message"=w438, "Element Name"="UNIT", "refs"=w436) -> ("Missing Element? (error)"=w437:bool)  [unwired: 7 in]
              }
              frame Enabled {
              }
            }
          }
          frame "_UNIT_SAMPLE" {
            n156 = for {
              tunnel: w451 -> [w459]
              tunnel: w450 -> [w458]
              tunnel: w449 -> [w457] mode=indexing
              tunnel: [w456] -> w447
              (unwired) T9[] [enum."UN_WT", enum."UN_WL%d"] items=["UN_VLV%d", "UN_PMP%d", "UN_WL%d", "UN_PH", "UN_EC", "UN_ORP", "UN_WT", "UN_PH2", "UN_ALFA1", "UN_BETA1", "UN_ALFA2", "UN_BETA2", "UN_ACID", "UN_BASE", "UN_WATER", "UN_ORPMIX"]
              n157 = Match Pattern(string=w457, regular expression="=") -> (before substring=w453:string, after substring=w454:string)  [unwired: 1 in, 2 out]
              n158 = case shown="\"UN_EC\", \"UN_ORP\", \"UN_PH\"" w453 {
                selector: w453 -> [w460 w474]
                tunnel: w459 -> [w469 w483]
                tunnel: w458 -> [w468 w482]
                tunnel: [w467 w481] -> w456
                tunnel: w454 -> [w461 w475]
                tunnel: string[] ["UN_WL", "UN_WT"] ("regular expression") -> [_ w473]
                frame "UN_EC", "UN_ORP", "UN_PH" {
                  n159 = call <vilib>:"Space Constant.vi"() -> ("String"=w463:string)
                  n160 = Match Pattern(string=w461, regular expression=w463) -> (after substring=w464:string)  [unwired: 1 in, 3 out]
                  n161 = case shown="\"ALARM\"" w464 {
                    tunnel: [type.nrt.elment-state."In Range" ("Enum 2") type.nrt.elment-state."Alarm" ("Enum 2") type.nrt.elment-state."Out of Range" ("Enum 2")] -> w462
                    frame "RANGE", Default {
                    }
                    frame "ALARM" {
                    }
                    frame "HIGH", "LOW" {
                    }
                  }
                  n162 = Select(t=type.nrt.elment-state."Alarm" ("Enum"), s=w468, f=w462) -> (s? t:f=w465:T6)
                  n163 = call "ntr.flow-panel.set-ref.vi"("Enum"=w465, "String Message"=w461, "Element Name"=w460, "refs"=w469) -> ("Missing Element? (error)"=w467:bool)  [unwired: 7 in]
                }
                frame Default {
                  n164 = call <vilib>:"Space Constant.vi"() -> ("String"=w477:string)
                  n165 = Match Pattern(string=w475, regular expression=w477) -> (after substring=w478:string)  [unwired: 1 in, 3 out]
                  n166 = case shown="\"RANGE\", Default" w478 {
                    tunnel: [type.nrt.elment-state."In Range" ("Enum 2") type.nrt.elment-state."Alarm" ("Enum 2") type.nrt.elment-state."Out of Range" ("Enum 2")] -> w476
                    frame "RANGE", Default {
                    }
                    frame "ALARM" {
                    }
                    frame "HIGH", "LOW" {
                    }
                  }
                  n167 = Select(t=type.nrt.elment-state."Alarm" ("Enum"), s=w482, f=w476) -> (s? t:f=w479:T6)
                  n168 = for {
                    tunnel: w483 -> [w492]
                    tunnel: [w491] -> w481
                    tunnel: w479 -> [w490]
                    tunnel: w475 -> [w486]
                    tunnel: w474 -> [w489]
                    tunnel: w473 -> [w488] mode=indexing
                    n169 = call <vilib>:"Space Constant.vi"() -> ("String"=w485:string)
                    n170 = Match Pattern(string=w486, regular expression=w485) -> (after substring=w484:string)  [unwired: 1 in, 3 out]
                    n171 = Match Pattern(string=w489, regular expression=w488) -> (match substring=w487:string)  [unwired: 1 in, 3 out]
                    n172 = case shown="\"0\", Default" w487 {
                      tunnel: w492 -> [_ w497 w502]
                      tunnel: [_ w496 w501] -> w491
                      tunnel: w490 -> [_ w495 w500]
                      tunnel: w486 -> [_ _ w499]
                      tunnel: w484 -> [_ w493 _]
                      frame "0", Default {
                      }
                      frame "UN_WL" {
                        n173 = call "ntr.flow-panel.set-ref.vi"("Enum"=w495, "String Message"=w493, "Element Name"="W_LEVEL", "refs"=w497) -> ("Missing Element? (error)"=w496:bool)  [unwired: 7 in]
                      }
                      frame "UN_WT" {
                        n174 = call "ntr.flow-panel.set-ref.vi"("Enum"=w500, "String Message"=w499, "Element Name"="W_TEMP", "refs"=w502) -> ("Missing Element? (error)"=w501:bool)  [unwired: 7 in]
                      }
                    }
                  }
                }
              }
            }
          }
          frame "_WASH_IN", "_WASH_OUT" {
            n175 = Index Array(array=w512) -> (element=w511:string)  [unwired: 1 in]
            n176 = String Subset(string=w508, offset (0)=1) -> (substring=w506:string)  [unwired: 1 in]
            n177 = Match Pattern(string=w511, regular expression="_") -> (after substring=w509:string)  [unwired: 1 in, 3 out]
            n178 = Select(t=type.nrt.elment-state."Alarm" ("Enum"), s=w516, f=type.nrt.elment-state."In Range" ("Enum")) -> (s? t:f=w513:T6)
            n179 = call "ntr.flow-panel.set-ref.vi"("Enum"=w513, "String Message"=w509, "Element Name"=w506, "refs"=w517) -> ()  [unwired: 7 in, 1 out]
          }
          frame Default {
          }
        }
        "State(Element)" <- w289
        "Missing Element?" <- w282
      }
    }
  }
